vi "Traps-10-06-2017.vi"(0 "d0Trap1":fxp<+/-,18,18> format="%.16g", 1 "heizenTrap1":bool, 2 "U_SPTrap1":fxp<+/-,26,5> format="%.23g", 3 "->Register":u32, 5 "d1Trap1":fxp<+/-,21,21> format="%.16g", 7 "Warten(uSec)":u16=5000, 9 "d0Trap2":fxp<+/-,18,18> format="%.16g", 11 "d1Trap2":fxp<+/-,21,21> format="%.16g", 12 "heizenTrap2":bool, 13 "U_SPTrap2":fxp<+/-,26,5> format="%.23g") -> (4 "U_MWTrap1":fxp<+/-,26,5> format="%.23g", 14 "Register->":u32, 15 "U_MWTrap2":fxp<+/-,26,5> format="%.23g")   [LabVIEW 2017]
uses:
  <vilib>/rvi/FXPMathLib/FxpDiv/subVIs/nifxpmath_Div_SimConfig.ctl
  <vilib>/rvi/eio/common/nirviEmuTemplateMethod_errors.vi
  <vilib>/rvi/FXPMathLib/FxpDiv/simVIs/DllFxpDivTemp_sub.vi
  <vilib>/eio/EIONode/EIONode.xnode
  <vilib>/rvi/FXPMathLib/FxpAdd/XNode/nifxpmath_Add.xnode
  <vilib>/rvi/FXPMathLib/FxpDiv/XNode/nifxpmath_Div.xnode
  <vilib>/rvi/FXPMathLib/FxpSub/XNode/nifxpmath_Sub.xnode
  <vilib>/rvi/FXPMathLib/FxpMul/XNode/nifxpmath_Multiplier.xnode
  <vilib>/rvi/FXPMathLib/sim/FxpSim.dll
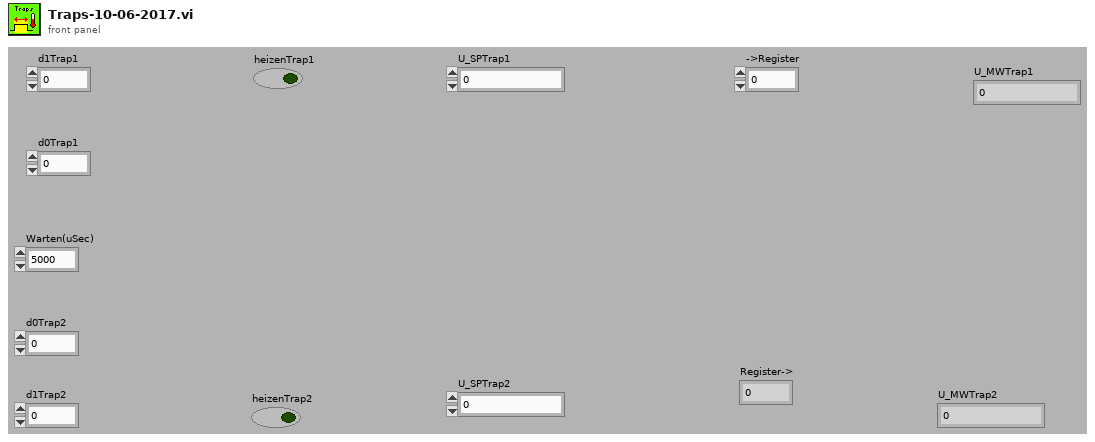
[diagram p1: front panel]
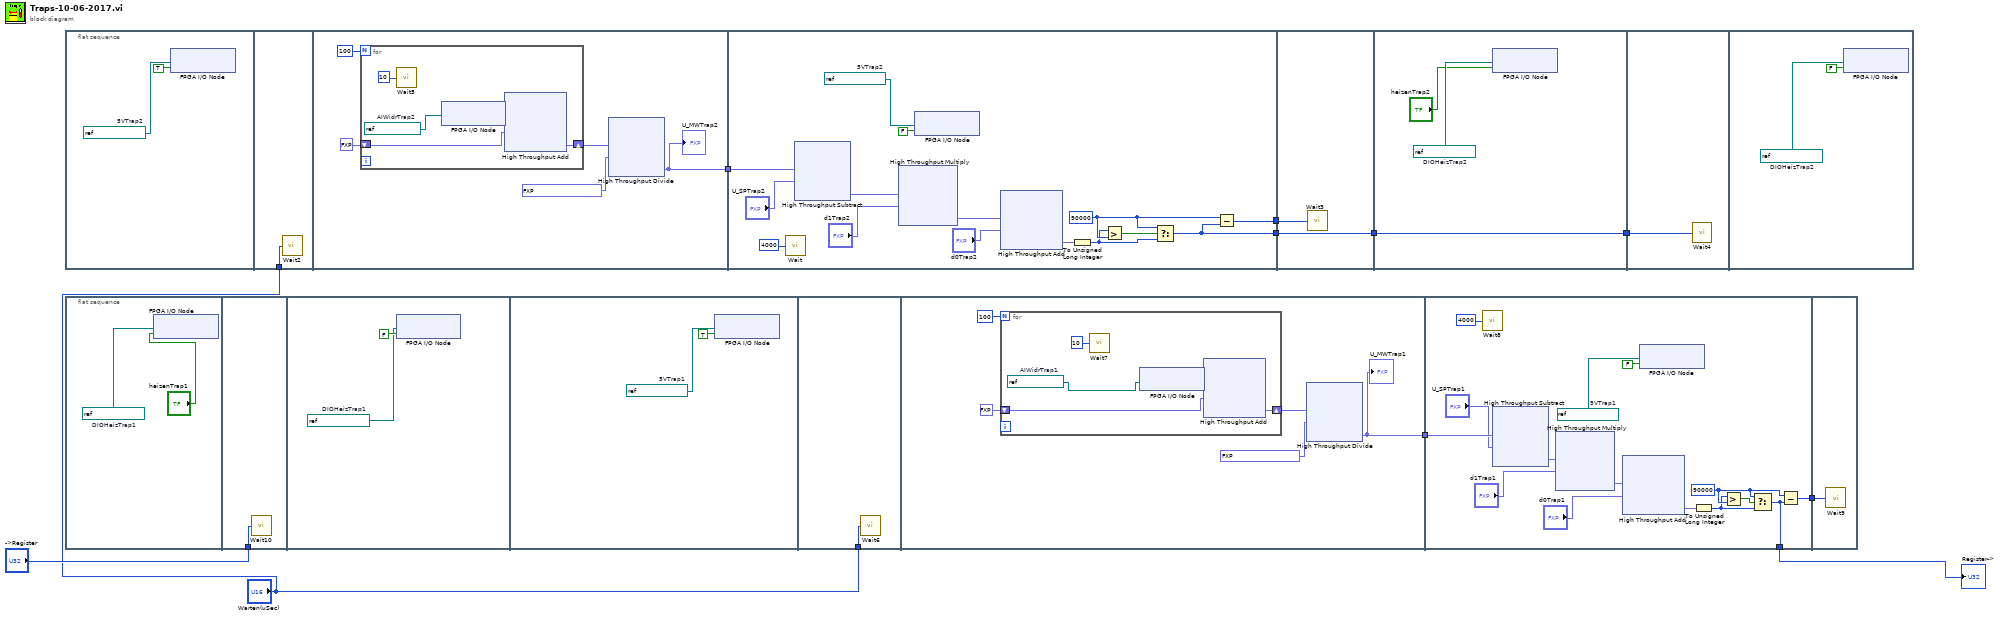
[diagram p0: block diagram]
diagram:
  n1 = flat-sequence {
    tunnel: "Warten(uSec)" -> [w13]
    tunnel: [w14] -> w9
    tunnel: w9 -> [w63]
    tunnel: [w55] -> w8
    tunnel: [w59] -> w7
    tunnel: [w67] -> w6
    tunnel: w8 -> [w67]
    tunnel: w7 -> [w66]
    tunnel: [w70] -> w5
    tunnel: w6 -> [w70]
    tunnel: w5 -> [w71]
    frame #0 {
      w11 = refnum<k21> "Mod6/DIO20"  # 5VTrap2
      n2 = xnode "FPGA I/O Node"("I/O-Objekt"=TRUE ("I/O Item"), "FPGA-I/O (Eingang)"=w11) -> ()  [unwired: 1 out]
    }
    frame #1 {
      n3 = call "Wait2"("Count(uSec)"=w13) -> ()  [unwired: 1 out]
    }
    frame #2 {
      n4 = for {
        N: 100 -> [_]
        shift-right: [w47] -> w18
        shift-left: fxp<+/-,33,12> 0.0 ("x+y") -> [w48]
        w46 = refnum<k21> "Mod1/AI31"  # AIWidrTrap2
        n5 = call "Wait5"("Count(uSec)"=u8 10) -> ()  [unwired: 1 out]
        n6 = xnode "FPGA I/O Node"("FPGA-I/O (Eingang)"=w46) -> ("I/O-Objekt"=w49:fxp<+/-,26,5>)  [unwired: 1 out]
        n7 = xnode "High Throughput Add"("x"=w49, "y"=w48) -> ("x+y"=w47:fxp<+/-,33,12>)
      }
      n8 = xnode "High Throughput Divide"("x"=w18, "y"=fxp<+/-,8,8> 100.0) -> ("x/y"=w14:fxp<+/-,26,5>)
      "U_MWTrap2" <- w14
    }
    frame #3 {
      w54 = refnum<k21> "Mod6/DIO20"  # 5VTrap2
      w57 = u32 90000 ("x")
      n9 = call "Wait"("Count(uSec)"=u16 4000) -> ()  [unwired: 1 out]
      n10 = xnode "High Throughput Subtract"("x"=w63, "y"="U_SPTrap2") -> ("x-y"=w62:fxp<+/-,26,5>)
      n11 = xnode "High Throughput Multiply"("x"=w62, "y"="d1Trap2") -> ("x*y"=w61:fxp<+/-,18,18>)
      n12 = xnode "FPGA I/O Node"("I/O-Objekt"=FALSE ("I/O Item"), "FPGA-I/O (Eingang)"=w54) -> ()  [unwired: 1 out]
      n13 = xnode "High Throughput Add"("x"=w61, "y"="d0Trap2") -> ("x+y"=w60:fxp<+/-,18,18>)
      n14 = To Unsigned Long Integer(number=w60) -> (unsigned 32bit integer=w56:u32)
      n15 = Greater?(x=w56, y=w57) -> (0:w58:bool)
      n16 = Select(t=w57, s=w58, f=w56) -> (s? t:f=w55:u32)
      n17 = Subtract(x=w57, y=w55) -> (x-y=w59:u32)
    }
    frame #4 {
      n18 = call "Wait3"("Count(uSec)"=w66) -> ()  [unwired: 1 out]
    }
    frame #5 {
      w69 = refnum<k21> "Mod6/DIO18"  # DIOHeizTrap2
      n19 = xnode "FPGA I/O Node"("I/O-Objekt"="heizenTrap2", "FPGA-I/O (Eingang)"=w69) -> ()  [unwired: 1 out]
    }
    frame #6 {
      n20 = call "Wait4"("Count(uSec)"=w71) -> ()  [unwired: 1 out]
    }
    frame #7 {
      w72 = refnum<k21> "Mod6/DIO18"  # DIOHeizTrap2
      n21 = xnode "FPGA I/O Node"("I/O-Objekt"=FALSE ("I/O Item"), "FPGA-I/O (Eingang)"=w72) -> ()  [unwired: 1 out]
    }
  }
  n22 = flat-sequence {
    tunnel: "->Register" -> [w76]
    tunnel: "Warten(uSec)" -> [w81]
    tunnel: [w82] -> w4
    tunnel: w4 -> [w131]
    tunnel: [w127] -> w3
    tunnel: [w123] -> w2
    tunnel: w3 -> [w134]
    frame #0 {
      w75 = refnum<k21> "Mod6/DIO19"  # DIOHeizTrap1
      n23 = xnode "FPGA I/O Node"("I/O-Objekt"="heizenTrap1", "FPGA-I/O (Eingang)"=w75) -> ()  [unwired: 1 out]
    }
    frame #1 {
      n24 = call "Wait10"("Count(uSec)"=w76) -> ()  [unwired: 1 out]
    }
    frame #2 {
      w77 = refnum<k21> "Mod6/DIO19"  # DIOHeizTrap1
      n25 = xnode "FPGA I/O Node"("I/O-Objekt"=FALSE ("I/O Item"), "FPGA-I/O (Eingang)"=w77) -> ()  [unwired: 1 out]
    }
    frame #3 {
      w79 = refnum<k21> "Mod6/DIO21"  # 5VTrap1
      n26 = xnode "FPGA I/O Node"("I/O-Objekt"=TRUE ("I/O Item"), "FPGA-I/O (Eingang)"=w79) -> ()  [unwired: 1 out]
    }
    frame #4 {
      n27 = call "Wait6"("Count(uSec)"=w81) -> ()  [unwired: 1 out]
    }
    frame #5 {
      n28 = for {
        N: 100 -> [_]
        shift-right: [w115] -> w86
        shift-left: fxp<+/-,33,12> 0.0 ("x+y") -> [w116]
        w114 = refnum<k21> "Mod1/AI30"  # AIWidrTrap1
        n29 = call "Wait7"("Count(uSec)"=u8 10) -> ()  [unwired: 1 out]
        n30 = xnode "FPGA I/O Node"("FPGA-I/O (Eingang)"=w114) -> ("I/O-Objekt"=w117:fxp<+/-,26,5>)  [unwired: 1 out]
        n31 = xnode "High Throughput Add"("x"=w117, "y"=w116) -> ("x+y"=w115:fxp<+/-,33,12>)
      }
      n32 = xnode "High Throughput Divide"("x"=w86, "y"=fxp<+/-,8,8> 100.0) -> ("x/y"=w82:fxp<+/-,26,5>)
      "U_MWTrap1" <- w82
    }
    frame #6 {
      w122 = refnum<k21> "Mod6/DIO21"  # 5VTrap1
      w125 = u32 90000 ("x")
      n33 = call "Wait8"("Count(uSec)"=u16 4000) -> ()  [unwired: 1 out]
      n34 = xnode "High Throughput Subtract"("x"=w131, "y"="U_SPTrap1") -> ("x-y"=w130:fxp<+/-,26,5>)
      n35 = xnode "High Throughput Multiply"("x"=w130, "y"="d1Trap1") -> ("x*y"=w129:fxp<+/-,18,18>)
      n36 = xnode "High Throughput Add"("x"=w129, "y"="d0Trap1") -> ("x+y"=w128:fxp<+/-,18,18>)
      n37 = xnode "FPGA I/O Node"("I/O-Objekt"=FALSE ("I/O Item"), "FPGA-I/O (Eingang)"=w122) -> ()  [unwired: 1 out]
      n38 = To Unsigned Long Integer(number=w128) -> (unsigned 32bit integer=w124:u32)
      n39 = Greater?(x=w124, y=w125) -> (0:w126:bool)
      n40 = Select(t=w125, s=w126, f=w124) -> (s? t:f=w123:u32)
      n41 = Subtract(x=w125, y=w123) -> (x-y=w127:u32)
    }
    frame #7 {
      n42 = call "Wait9"("Count(uSec)"=w134) -> ()  [unwired: 1 out]
    }
  }
  "Register->" <- w2
